vi "Test Helper Loop Stopped on Process Stop.vi"(8 "error in (no error)":errorcluster, 11 "Helper Loop Test In":refnum<class "Helper Loop Test.lvclass">) -> (0 "error out":errorcluster, 3 "Helper Loop Test Out":refnum<class "Helper Loop Test.lvclass">)   [LabVIEW 2020, in "Helper Loop Test.lvclass"]
uses:
  Helper Loop Test.lvclass
  C:/Program Files (x86)/National Instruments/LabVIEW 2020/vi.lib/Astemes/LUnit/Test Case.lvclass
  source/Framework Test Suite/Mock Process/Mock Process.lvclass
  C:/git/astemes-triarc-framework/source/Framework/Process/Process.lvclass
  source/Framework/Process/Process.lvclass/Process.ctl
  <vilib>/Astemes/LUnit/Test Case.lvclass/Test Case.ctl
  cf682f82-6362-4fa3-93a3-bc290b111215.vi
  source/Framework/Process/Public/Lifecycle/Get Lifecycle State.vi
  source/Framework/Process/Private/SubVIs/Wait for finish.vi
  source/Framework/Process/Private/SubVIs/Set Lifecycle State.vi
  source/Framework/Process/Protected/Messaging/Send Message.vi
  source/Framework/Broadcast Event Helpers/Execution timer.vi
  <vilib>/Astemes/LUnit/Append Pass Result.vi
  <vilib>/Astemes/LUnit/Append Fail Result.vi
  <vilib>/Astemes/LUnit/Describe Comparison.vi
  <vilib>/Astemes/LUnit/Compare Variants.vi
  <vilib>/Utility/error.llb/Clear Errors.vi
  source/Framework/Process/Private/SubVIs/Handle Debug Data.vi
  source/Framework/Logging/Log Debug.vi
  <vilib>/AdvancedString/1D String Array to Delimited String.vi
  <vilib>/Utility/High Resolution Relative Seconds.vi
  <vilib>/Utility/error.llb/Error Cluster From Error Code.vi
  source/Framework/Process/Public/Read Name.vi
  source/Framework/Broadcast Event Dequeuers/Dequeue Broadcast Message.vi
  <vilib>/Astemes/LUnit/Describe Variant.vi
  source/Framework/Callback/Callback.lvclass
  source/Framework/Process/Process.lvclass
  source/Framework/Broadcast Event Helpers/Broadcast Event Helpers.lvlib
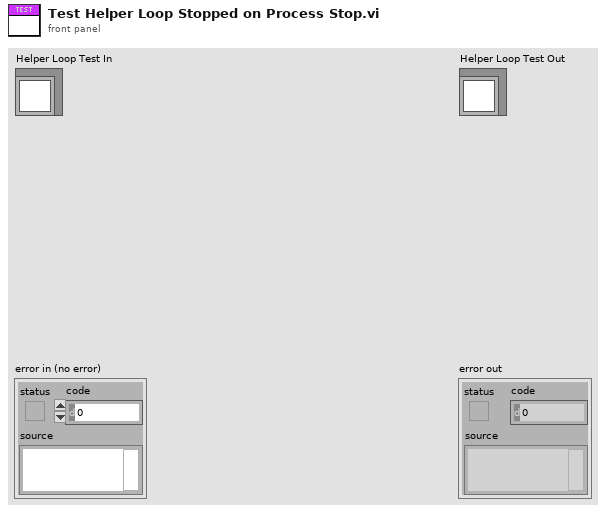
[diagram p1: front panel]
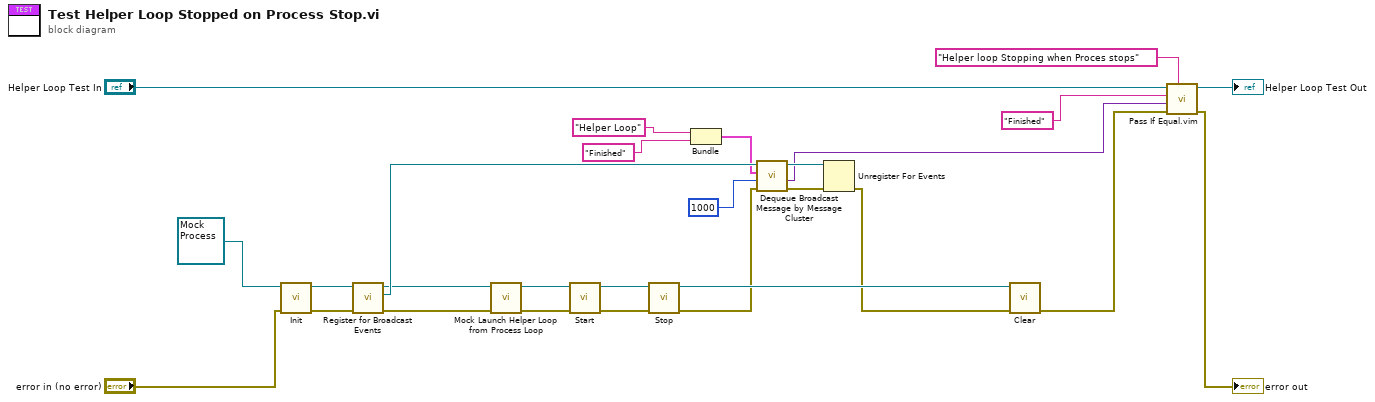
[diagram p0: block diagram]
diagram:
  n1 = call-dynamic "Init.vi"("error in (no error)"="error in (no error)", "Mock Process In"=refnum<class "Mock Process.lvclass"> refnum) -> ("error out"=w26:errorcluster, "Mock Process Out"=w27:refnum<class "Mock Process.lvclass">)  [unwired: 8 in]
  n2 = call "Register for Broadcast Events.vi"("error in (no error)"=w26, "Process In"=w27) -> ("error out"=w25:errorcluster, "Event Registration Refnum Out"=w17:refnum<event-registration>, "Process Out"=w4:refnum<class "Mock Process.lvclass">)  [unwired: 7 in]
  n3 = call "Mock Launch Helper Loop from Process Loop.vi"("error in (no error)"=w25, "Mock Process in"=w4) -> ("error out"=w5:errorcluster, "Mock Process out"=w2:refnum<class "Mock Process.lvclass">)  [unwired: 8 in]
  n4 = call "Start.vi"("error in (no error)"=w5, "Process In"=w2) -> ("error out"=w3:errorcluster, "Process Out"=w1:refnum<class "Mock Process.lvclass">)  [unwired: 7 in, 1 out]
  n5 = call "Stop.vi"("error in (no error)"=w3, "Process In"=w1) -> ("error out"=w15:errorcluster, "Process Out"=w24:refnum<class "Mock Process.lvclass">)  [unwired: 7 in, 1 out]
  n6 = Bundle("y"="Helper Loop", "Description"="Finished") -> (w6:cluster{"y":string, "Description":string})  [unwired: 1 in]
  n7 = call "Dequeue Broadcast Message by Message Cluster.vi"("error in (no error)"=w15, "Timeout (-1)"=1000, "Message"=w6, "Event Registration Refnum"=w17) -> ("error out"=w11:errorcluster, "Message Data"=w10:variant, "Event Registration Refnum Out"=w12:refnum<event-registration>)  [unwired: 3 in, 2 out]
  n8 = Unregister For Events(event registration refnum=w12, error in=w11) -> (error out=w14:errorcluster)
  n9 = call-dynamic "Clear.vi"("error in (no error)"=w14, "Mock Process In"=w24) -> ("error out"=w23:errorcluster)  [unwired: 9 in]
  n10 = call "Pass If Equal.vim"("Description"="Helper loop Stopping when Proces stops", "error in (no error)"=w23, "Actual"=w10, "Expected"="Finished" ("Description"), "LUnit Test Case In"="Helper Loop Test In") -> ("error out"=→"error out":errorcluster, "LUnit Test Case Out"=→"Helper Loop Test Out":refnum<class "Helper Loop Test.lvclass">)  [unwired: 5 in]
